vi "adder_example.vi"() -> ()   [LabVIEW 2018]
uses:
  C:/Users/booko/Desktop/ENABLE/UpDownCounter/bin/Debug/netstandard2.0/UpDownCounter.dll
  UpDownCounter/bin/Debug/netstandard2.0/UpDownCounter.dll
panel:
  in  "error in (no error)":errorcluster
  out "error out":errorcluster
  out "adder":dbl
  in  "y":dbl
  in  "x":dbl
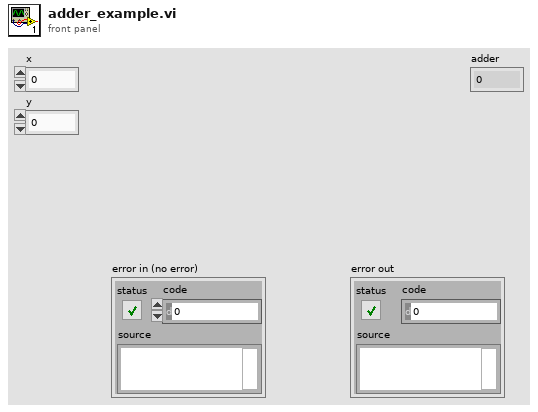
[diagram p1: front panel]
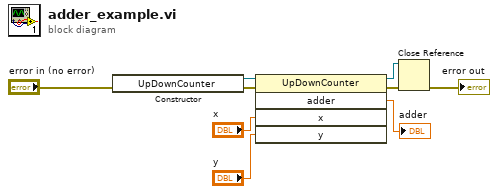
[diagram p0: block diagram]
diagram:
  n1 = constructor class="UpDownCounter"(error in="error in (no error)") -> (reference out=w9:refnum<k24>, error out=w4:errorcluster)  [unwired: 2 in, 1 out]
  n2 = invoke class="UpDownCounter" method="adder"(reference=w9, error in=w4, "x"="x", "y"="y") -> (reference out=w5:refnum<k24>, error out=w3:errorcluster, "adder"=→"adder":dbl)  [unwired: 1 in, 2 out]
  n3 = Close Reference(reference=w5, error in (no error)=w3) -> (error out=→"error out":errorcluster)
